vi "Apply Gripper Motor Limits.vi"(8 "error in (no error)":errorcluster, 11 "KUKA youBot gripper in":refnum<class "NI_Robotics_KUKA youBot Gripper.lvclass">) -> (0 "error out":errorcluster, 3 "KUKA youBot gripper out":refnum<class "NI_Robotics_KUKA youBot Gripper.lvclass">)   [LabVIEW 2017, in "NI_Robotics_KUKA youBot Host.lvlib" / "NI_Robotics_KUKA youBot Gripper.lvclass"]
uses:
  <vilib>/robotics/KUKA youBot/Basic Device/Gripper/NI_Robotics_KUKA youBot Gripper.lvclass
  <vilib>/robotics/KUKA youBot/Basic Device/Gripper/NI_Robotics_KUKA youBot Gripper.lvclass/NI_Robotics_KUKA youBot Gripper.ctl
  <vilib>/robotics/KUKA youBot/Motor/Gripper Motor/NI_Robotics_KUKA youBot Gripper Motor.lvclass
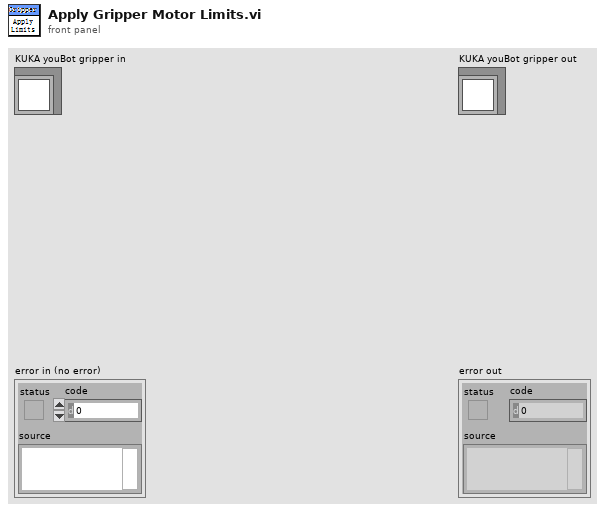
[diagram p1: front panel]
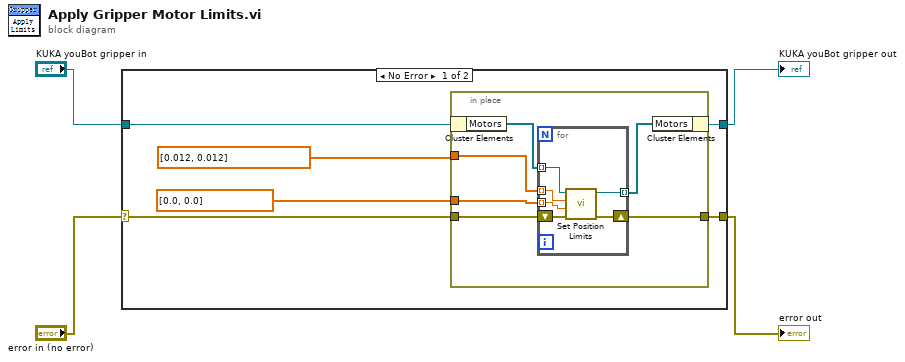
[diagram p0: block diagram]
diagram:
  n1 = case shown="No Error" "error in (no error)" {
    selector: "error in (no error)" -> [w9 w23]
    tunnel: [w8 w23] -> w2
    tunnel: [w7 w24] -> w1
    tunnel: "KUKA youBot gripper in" -> [w10 w24]
    frame No Error {
      n2 = in-place {
        in-place-border: w9 -> [w14]
        in-place-border: [w13] -> w8
        in-place-border: dbl[] [0.012, 0.012] -> [w12]
        in-place-border: dbl[] [0.0, 0.0] -> [w11]
        n3 = in-place-cluster #1(w10) -> ("Motors"=w16:refnum<class "NI_Robotics_KUKA youBot Gripper Motor.lvclass">[])
        n4 = for {
          tunnel: w16 -> [w19] mode=indexing
          tunnel: [w20] -> w15 mode=indexing
          shift-right: [w21] -> w13
          shift-left: w14 -> [w22]
          tunnel: w12 -> [w18] mode=indexing
          tunnel: w11 -> [w17] mode=indexing
          n5 = call <vilib>:"Set Position Limits.vi"("error in (no error)"=w22, "min dist (m)"=w17, "max dist (m)"=w18, "KUKA youBot gripper motor in"=w19) -> ("error out"=w21:errorcluster, "KUKA youBot gripper motor out"=w20:refnum<class "NI_Robotics_KUKA youBot Gripper Motor.lvclass">)  [unwired: 6 in]
        }
        n6 = in-place-cluster #1("Motors"=w15) -> (w7:refnum<class "NI_Robotics_KUKA youBot Gripper.lvclass">)
      }
    }
    frame Error {
    }
  }
  "error out" <- w2
  "KUKA youBot gripper out" <- w1
